vi "Image Capacity.vi"(11 "image data":T1) -> (3 "Capacity Bytes":i32)   [LabVIEW 2020]
uses:
  <vilib>/picture/picture.llb/imagedata.ctl
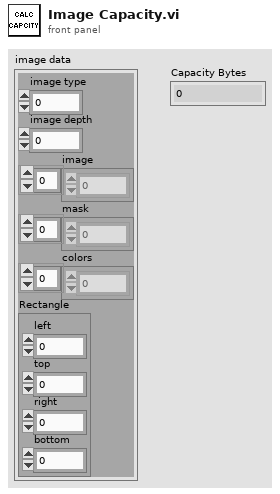
[diagram p1: front panel]
types:
  T1 = typedef "imagedata.ctl" = cluster{"image type":i32, "image depth":i32, "image":u8[], "mask":u8[], "colors":u32[], "Rectangle":cluster{"left":i16, "top":i16, "right":i16, "bottom":i16}}
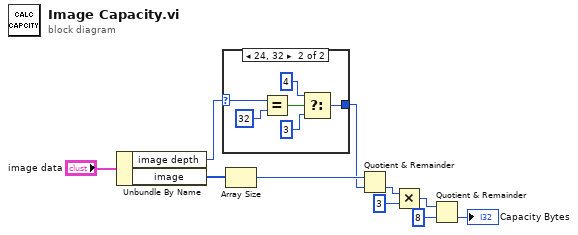
[diagram p0: block diagram]
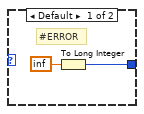
[diagram p2: hidden frame]
diagram:
  n1 = Unbundle By Name("image data") -> ("image depth"=w9:i32, "image"=w8:u8[])
  n2 = case shown="24, 32" w9 {
    selector: w9 -> [_ w18]
    tunnel: [w11 w13] -> w6
    frame Default {
      # "#ERROR"
      n3 = To Long Integer(number=inf) -> (32bit integer=w11:i32)
    }
    frame 24, 32 {
      n4 = Equal?(x=w18, y=32) -> (x = y?=w16:bool)
      n5 = Select(t=4, s=w16, f=3) -> (s? t:f=w13:i32)
    }
  }
  n6 = Array Size(array=w8) -> (size(s)=w7:i32)
  n7 = Quotient & Remainder(x=w7, y=w6) -> (floor(x/y)=w5:i32)  [unwired: 1 out]
  n8 = Multiply(x=w5, y=3) -> (x*y=w3:i32)
  n9 = Quotient & Remainder(x=w3, y=8) -> (floor(x/y)=→"Capacity Bytes":i32)  [unwired: 1 out]
